vi "数据发送处理.vi"(1 "PWM":dbl) -> (0 "字符串":string)   [LabVIEW 2022 SP3]
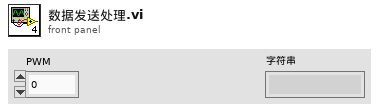
[diagram p1: front panel]
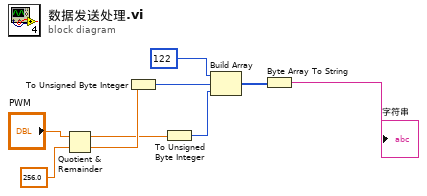
[diagram p0: block diagram]
diagram:
  n1 = Quotient & Remainder(x="PWM", y=256.0) -> (x-y*floor(x/y)=w4:dbl, floor(x/y)=w5:dbl)
  n2 = To Unsigned Byte Integer(number=w5) -> (unsigned 8bit integer=w8:u8)
  n3 = To Unsigned Byte Integer(number=w4) -> (unsigned 8bit integer=w3:u8)
  n4 = Build Array(u8 122, w8, w3) -> (w2:u8[])
  n5 = Byte Array To String(unsigned byte array=w2) -> (string=→"字符串":string)
